vi "WPI_CameraSend Images To PC Loop.vi"(8 "error in (no error)":errorcluster, 9 "port":u16=1181, 10 "IP CGI string":string="/axis-cgi/mjpg/video.cgi") -> ()   [LabVIEW 2018]
doc: "This VI is used to serve images from one or more named cameras on your robot to the dashboard, SmartDashboard, or compatible web browser. Camera name and type info is published using network tables. Connections are on port 1181 by default and the URL for streaming can be found by looking at the network \"camera\"/streams variable. Cameras that are opened and stored in the name registry are automatically published by that name.\n\nThis VI runs in parallel with other code and should be placed in Robot Main or in Periodic Tasks.\n\nThis software is licensed. Open the labview\\readme\\WPI Robotics Library Open Source License.txt file for more information."
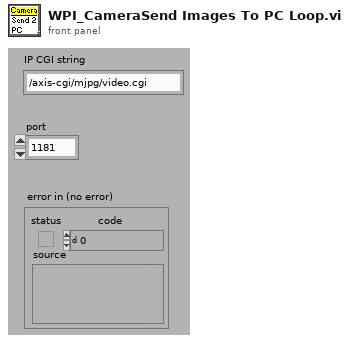
[diagram p1: front panel]
types:
  T1 = enum16{"Standard", "Buffered", "CRLF", "Immediate"}
  T2 = cluster{"token string":string, "token string 2":string}[]
  T3 = cluster{"Type":u32, "Version":u32, "Flags":u32, "SerialNumberHigh":u32, "SerialNumberLow":u32, "BusType":u32, "InterfaceName":string, "VendorName":string, "ModelName":string, "CameraFileName":string, "CameraAttributeURL":string}[]
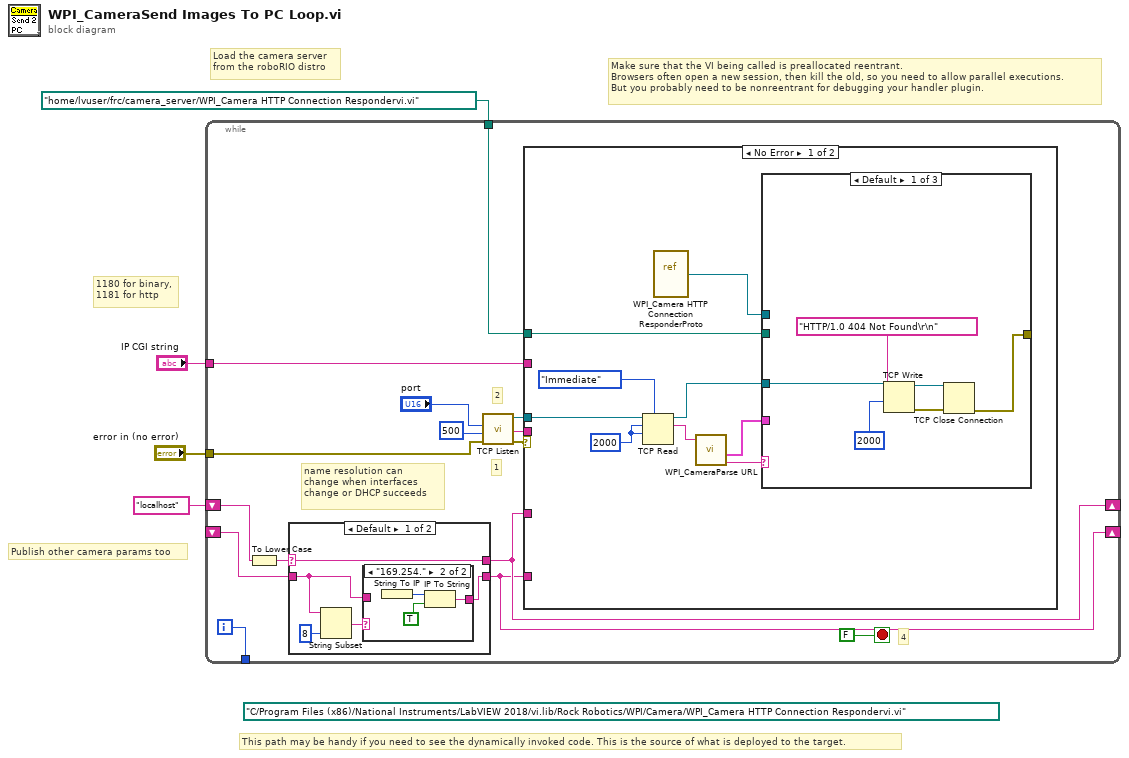
[diagram p0: block diagram]
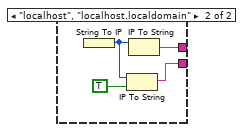
[diagram p3: hidden frame]
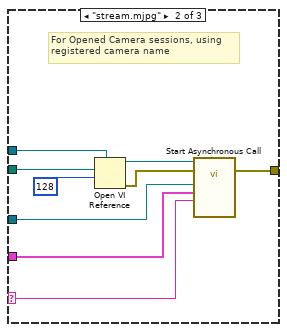
[diagram p4: hidden frame]
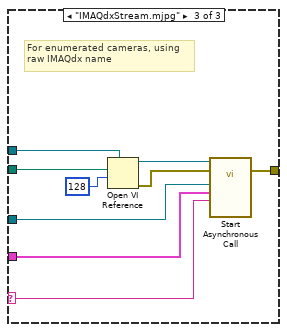
[diagram p5: hidden frame]
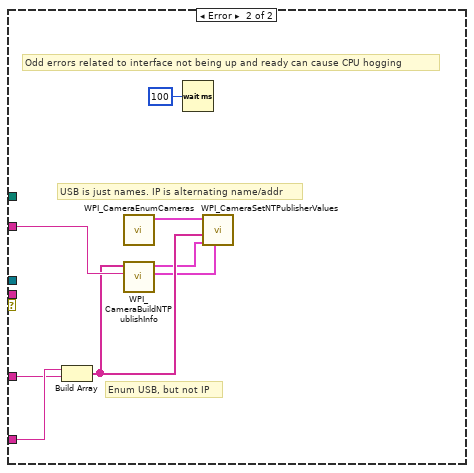
[diagram p6: hidden frame]
diagram:
  (unwired) path "C:/Program Files (x86)/National Instruments/LabVIEW 2018/vi.lib/Rock Robotics/WPI/Camera/WPI_Camera HTTP Connection Respondervi.vi"
  # "This path may be handy if you need to see the dynamically invoked code. This is the source of what is deployed to the target."
  # "Load the camera server\nfrom the roboRIO distro"
  # "Make sure that the VI being called is preallocated reentrant.\nBrowsers often open a new session, then kill the old, so you need to allow parallel executions.\nBut you probably need to be nonreentrant for debugging your handler plugin."
  # "Publish other camera params too"
  # "1180 for binary,\n1181 for http"
  n1 = while {
    tunnel: "error in (no error)" -> [w18]
    tunnel: [w13] -> _
    shift-right: [w9] -> _
    shift-left: "localhost" -> [w10]
    shift-right: [w7] -> _
    shift-left: _ -> [w8]
    tunnel: "IP CGI string" -> [w6]
    tunnel: path "/home/lvuser/frc/camera_server/WPI_Camera HTTP Connection Respondervi.vi" -> [w5]
    i -> [w13]
    stop <- FALSE ("status") stop-if-true
    # "name resolution can\nchange when interfaces\nchange or DHCP succeeds"
    # "4"
    # "1"
    # "2"
    n2 = To Lower Case(string=w10) -> (all lower case string=w11:string)
    n3 = case shown="Default" w11 {
      selector: w11 -> [w24 _]
      tunnel: [w24 w32] -> w9
      tunnel: w8 -> [w21 _]
      tunnel: [w20 w29] -> w7
      frame Default {
        n4 = String Subset(string=w21, length (rest)=8 ("length (rest)")) -> (substring=w22:string)  [unwired: 1 in]
        n5 = case shown="\"169.254.\"" w22 {
          tunnel: w21 -> [w25 _]
          tunnel: [w25 w26] -> w20
          frame Default {
          }
          frame "169.254." {
            n6 = String To IP() -> (0:w28:u32)  [unwired: 1 in]
            n7 = IP To String(1:TRUE ("dot notation? (F)"), 2:w28) -> (0:w26:string)
          }
        }
      }
      frame "localhost", "localhost.localdomain" {
        n8 = String To IP() -> (0:w30:u32)  [unwired: 1 in]
        n9 = IP To String(1:TRUE ("dot notation? (F)"), 2:w30) -> (0:w29:string)
        n10 = IP To String(2:w30) -> (0:w32:string)  [unwired: 1 in]
      }
    }
    n11 = call <vilib>:"TCP Listen.vi"("error in (no error)"=w18, "timeout ms (wait forever: -1)"=u16 500 ("port"), "port"="port") -> ("error out"=w15:errorcluster, "remote address"=w19:string, "connection ID"=w17:refnum<k5>)  [unwired: 1 in, 5 out]
    n12 = case shown="No Error" w15 {
      tunnel: w19 -> [_ _]
      tunnel: w17 -> [w39 _]
      tunnel: w9 -> [_ w71]
      tunnel: w7 -> [_ w72]
      tunnel: w6 -> [_ w70]
      tunnel: w5 -> [w33 _]
      frame No Error {
        w40 = 2000
        n13 = TCP Read(connection ID=w39, bytes to read=w40, 7:T1."Immediate" ("mode (standard)"), 9:w40) -> (connection ID out=w38:refnum<k5>, data out=w36:string)  [unwired: 1 in, 1 out]
        n14 = vi-ref <vilib>:"WPI_Camera HTTP Connection ResponderProto.vi"() -> (w34:refnum<vi>)
        n15 = call <vilib>:"WPI_CameraParse URL.vi"("URL"=w36) -> ("cgi string"=w35:string, "parameters"=w37:T2)  [unwired: 7 in, 2 out]
        n16 = case shown="Default" w35 {
          selector: w35 -> [_ w51 w58]
          tunnel: w33 -> [_ w56 w65]
          tunnel: w38 -> [w47 w55 w63]
          tunnel: [w42 w53 w61] -> _
          tunnel: w37 -> [_ w52 w60]
          tunnel: w34 -> [_ w50 w57]
          frame Default {
            n17 = TCP Write(connection ID=w47, data in="HTTP/1.0 404 Not Found\r\n" ("regular expression"), 9:2000) -> (connection ID out=w46:refnum<k5>, error out=w43:errorcluster)  [unwired: 1 in, 1 out]
            n18 = TCP Close Connection(connection ID=w46, error in (no error)=w43) -> (error out=w42:errorcluster)  [unwired: 2 out]
          }
          frame "stream.mjpg" {
            # "For Opened Camera sessions, using\nregistered camera name"
            n19 = Open VI Reference(type specifier VI Refnum (for type only)=w50, vi path=w56, options=128) -> (vi reference=w49:refnum<vi>, error out=w54:errorcluster)  [unwired: 3 in]
            n20 = call-by-ref "Start Asynchronous Call"(reference=w49, error in=w54, "CGI String"=w51, "parameters"=w52, "connection ID"=w55) -> (error out=w53:errorcluster)  [unwired: 9 in, 1 out]
          }
          frame "IMAQdxStream.mjpg" {
            # "For enumerated cameras, using\nraw IMAQdx name"
            n21 = Open VI Reference(type specifier VI Refnum (for type only)=w57, vi path=w65, options=128) -> (vi reference=w59:refnum<vi>, error out=w62:errorcluster)  [unwired: 3 in]
            n22 = call-by-ref "Start Asynchronous Call"(reference=w59, error in=w62, "CGI String"=w58, "parameters"=w60, "connection ID"=w63) -> (error out=w61:errorcluster)  [unwired: 9 in, 1 out]
          }
        }
      }
      frame Error {
        # "Enum USB, but not IP"
        # "USB is just names. IP is alternating name/addr"
        # "Odd errors related to interface not being up and ready can cause CPU hogging"
        n23 = Build Array(w72, w71) -> (w68:string[])
        n24 = call <vilib>:"WPI_CameraEnumCameras.vi"() -> ("USB Cams"=w69:T3)  [unwired: 10 in, 1 out]
        n25 = call <vilib>:"WPI_CameraBuildNTPublishInfo.vi"("IP CGI string"=w70, "RIO Addresses"=w68) -> ("Streams"=w66:cluster{string, "URLs":string[]}[], "Sources"=w67:cluster{string, string}[])  [unwired: 8 in]
        n26 = Wait (ms)(milliseconds to wait=u32 100) -> ()  [unwired: 1 out]
        n27 = call <vilib>:"WPI_CameraSetNTPublisherValues.vi"("Streams"=w66, "Sources"=w67, "roboRIO Addresses"=w68, "USB Cams"=w69) -> ()  [unwired: 8 in]
      }
    }
  }
